vi "Write Range.vi"(8 "error in (no error)":errorcluster, 10 "Range":T1, 11 "Scanner in":refnum<class "Scanner.lvclass">) -> (0 "error out":errorcluster, 2 "# Points":u32, 3 "Scanner out":refnum<class "Scanner.lvclass">)   [LabVIEW 2015, in "Scanner.lvclass"]
doc: "Set the Range of this Scanner to the Range of another Scanner."
uses:
  Scanner.lvclass
  Range.ctl
  Scanner.lvclass/Scanner.ctl
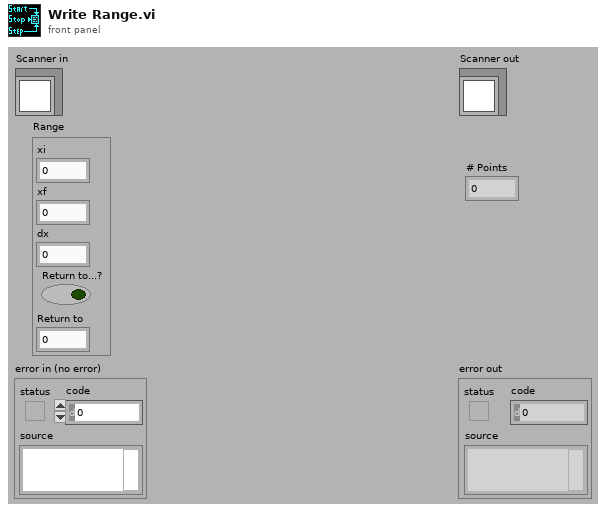
[diagram p1: front panel]
types:
  T1 = typedef "Scanner.lvclass/Range.ctl" = cluster{"xi":dbl, "xf":dbl, "dx":dbl, "Return to...?":bool, "Return to":dbl}
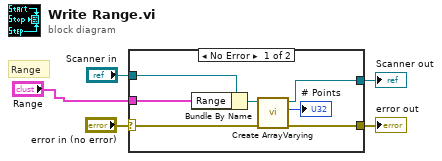
[diagram p0: block diagram]
diagram:
  # "Range"
  n1 = case shown="No Error" "error in (no error)" {
    selector: "error in (no error)" -> [w9 w14]
    tunnel: [w12 w14] -> w4
    tunnel: [w11 w13] -> w2
    tunnel: "Scanner in" -> [w7 w13]
    tunnel: "Range" -> [w6 _]
    frame No Error {
      n2 = Bundle By Name(cluster=w7, "Range"=w6) -> (w8:refnum<class "Scanner.lvclass">)
      n3 = call "Create ArrayVarying.vi"("error in (no error)"=w9, "Scanner.lvclass"=w8) -> ("error out"=w12:errorcluster, "# Points"=→"# Points":u32, "Scanner.lvclass out"=w11:refnum<class "Scanner.lvclass">)  [unwired: 7 out]
    }
    frame Error {
    }
  }
  "error out" <- w4
  "Scanner out" <- w2
